vi "close.vi"(8 "error in":errorcluster, 11 "Simple Sequencer TBM runtime in":refnum<class "Simple Sequencer TBM runtime.lvclass">) -> (0 "error out":errorcluster)   [LabVIEW 2015, in "Simple Sequencer TBM runtime.lvclass"]
doc: "Provides an interface for terminating a module instance. While this interface performs no operations, a child should close and deallocate any open references or memory."
uses:
  Simple Sequencer TBM runtime.lvclass
  Simple Sequencer TBM runtime.lvclass/Simple Sequencer TBM runtime.ctl
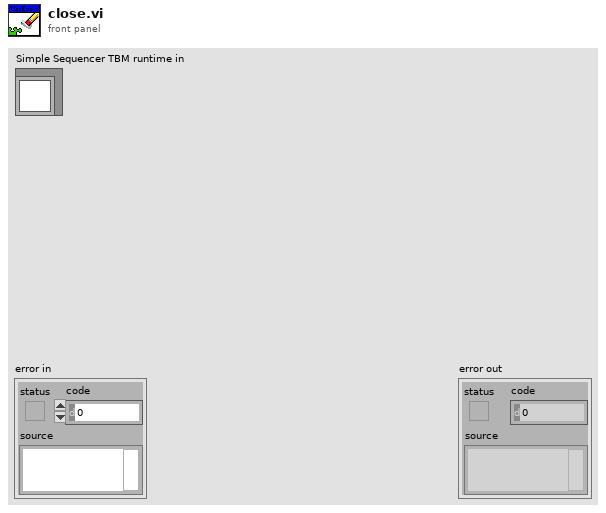
[diagram p1: front panel]
types:
  T1 = typedef "AMC.lvlib/Message Queue.ctl" = refnum<queue>
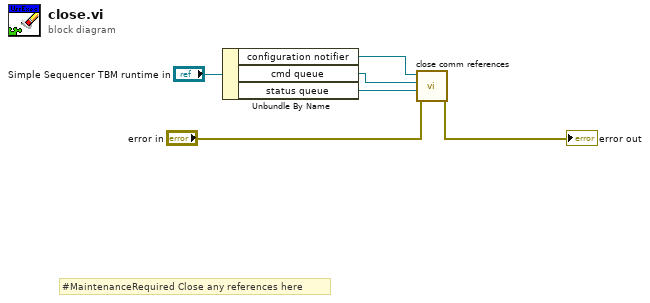
[diagram p0: block diagram]
diagram:
  # "#MaintenanceRequired Close any references here"
  n1 = Unbundle By Name("Simple Sequencer TBM runtime in") -> ("configuration notifier"=w3:refnum<notifier>, "cmd queue"=w2:T1, "status queue"=w1:T1)
  n2 = call "close comm references.vi"("error in (no error)"="error in", "status queue"=w1, "cmd queue"=w2, "configuration notifier"=w3) -> ("error out"=→"error out":errorcluster)  [unwired: 7 in]
